vi "PNG Write.vi"(8 "error in (no error)":errorcluster, 10 "Chunks":T1(array[cluster]) {"CRC" format="%08x"}, 11 "Image Path (*.png)":path) -> (0 "error out":errorcluster, 3 "dup Image Path":path)   [LabVIEW 2022 SP3, in "VI-Snippet.lvlib"]
doc: "Writes the PNG image chunks to the <b>Image Path (*.png)</b>."
uses:
  VI-Snippet.lvlib
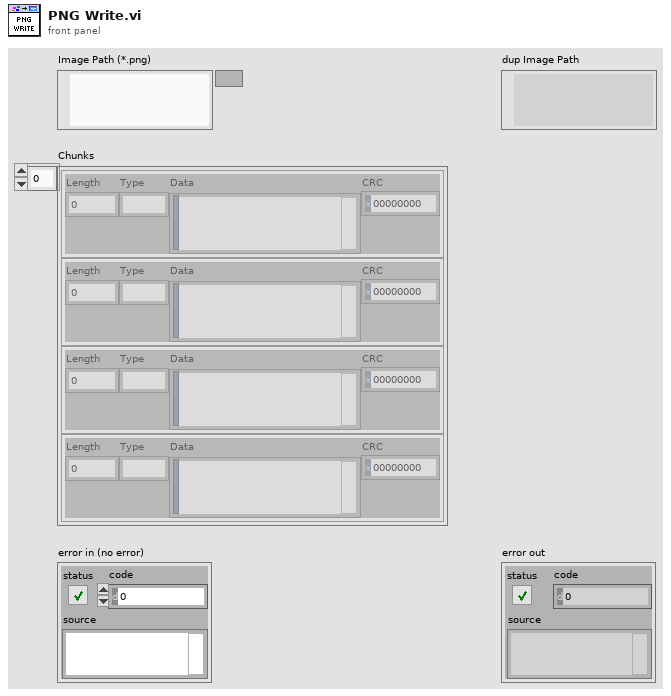
[diagram p1: front panel]
types:
  T1 = cluster{"Length":i32, "Type":string, "Data":string, "CRC":u32}[]
  T2 = enum16{"open", "replace", "create", "open or create", "replace or create", "replace or create with confirmation"}
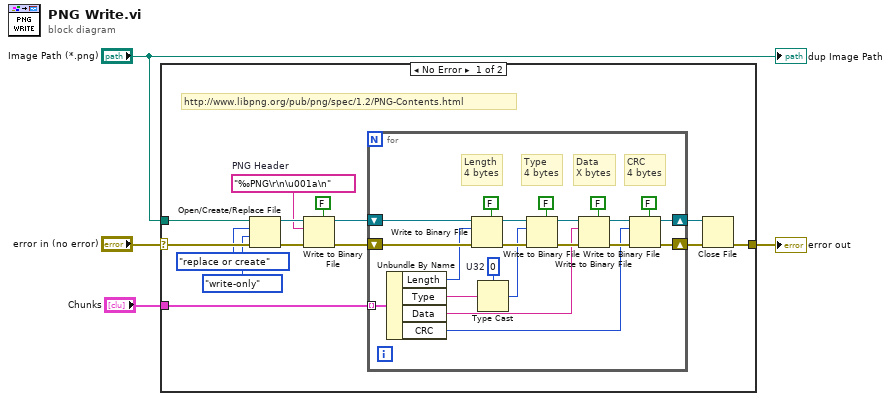
[diagram p0: block diagram]
diagram:
  n1 = case shown="No Error" "error in (no error)" {
    selector: "error in (no error)" -> [w18 w40]
    tunnel: "Image Path (*.png)" -> [w17 _]
    tunnel: [w14 w40] -> w3
    tunnel: "Chunks" -> [w6 _]
    frame No Error {
      w9 = "‰PNG\r\n\u001a\n"  # PNG Header
      # "http://www.libpng.org/pub/png/spec/1.2/PNG-Contents.html"
      n2 = Open/Create/Replace File(file path (use dialog)=w17, error in=w18, operation (0:open)=T2."replace or create", access (0:read/write)=enum16{"read/write", "read-only", "write-only"}."write-only") -> (refnum out=w16:refnum<file>, error out=w11:errorcluster)  [unwired: 2 in, 1 out]
      n3 = Write to Binary File(file (use dialog)=w16, data=w9, error in=w11, 5:FALSE ("prepend array or string size? (T)")) -> (refnum out=w8:refnum<file>, error out=w7:errorcluster)  [unwired: 2 in, 1 out]
      n4 = for {
        shift-right: [w20] -> w15
        shift-left: w7 -> [w36]
        tunnel: w6 -> [w39] mode=indexing
        shift-right: [w19] -> w13
        shift-left: w8 -> [w37]
        w30 = 0  # U32
        # "CRC\n4 bytes"
        # "Data\nX bytes"
        # "Type\n4 bytes"
        # "Length\n4 bytes"
        n5 = Unbundle By Name(w39) -> ("Length"=w35:i32, "Type"=w31:string, "Data"=w25:string, "CRC"=w21:u32)
        n6 = Write to Binary File(file (use dialog)=w37, data=w35, error in=w36, 5:FALSE ("prepend array or string size? (T)")) -> (refnum out=w32:refnum<file>, error out=w33:errorcluster)  [unwired: 2 in, 1 out]
        n7 = Type Cast(type=w30, x=w31) -> (*(type *) &x=w29:i32)
        n8 = Write to Binary File(file (use dialog)=w32, data=w29, error in=w33, 5:FALSE ("prepend array or string size? (T)")) -> (refnum out=w26:refnum<file>, error out=w27:errorcluster)  [unwired: 2 in, 1 out]
        n9 = Write to Binary File(file (use dialog)=w26, data=w25, error in=w27, 5:FALSE ("prepend array or string size? (T)")) -> (refnum out=w22:refnum<file>, error out=w23:errorcluster)  [unwired: 2 in, 1 out]
        n10 = Write to Binary File(file (use dialog)=w22, data=w21, error in=w23, 5:FALSE ("prepend array or string size? (T)")) -> (refnum out=w19:refnum<file>, error out=w20:errorcluster)  [unwired: 2 in, 1 out]
      }
      n11 = Close File(refnum=w13, error in=w15) -> (error out=w14:errorcluster)  [unwired: 1 out]
    }
    frame Error {
    }
  }
  "error out" <- w3
  "dup Image Path" <- "Image Path (*.png)"
